vi "Handle getAll.vi"(8 "error in (no error)":errorcluster, 11 "Temperhum":refnum<class "Instrument.Temperhum.lvclass">) -> (0 "error out":errorcluster, 2 "getAll":variant, 3 "Instrument.FrameworkTemplate out":refnum<class "Instrument.Temperhum.lvclass">)   [LabVIEW 2019, in "Instrument.Temperhum.lvclass"]
uses:
  Instrument.Temperhum.lvclass
  Typedefs/Instrument.Temperhum.getAll--Cluster.ctl
  Instrument.Temperhum.lvclass/Instrument.Temperhum.ctl
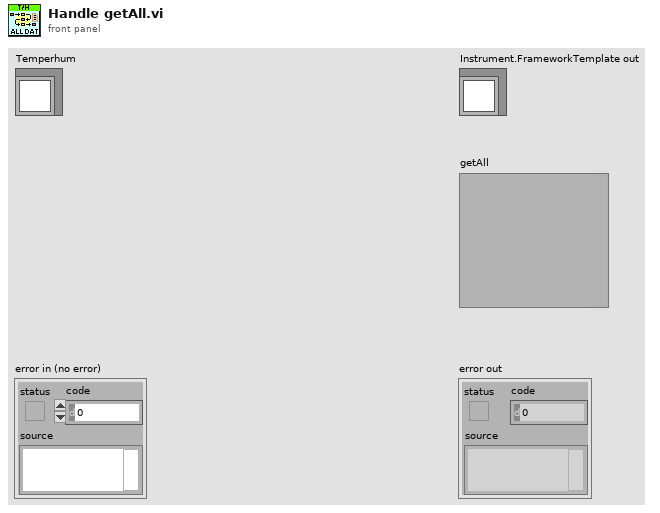
[diagram p1: front panel]
types:
  T1 = typedef "Instrument.Temperhum.lvclass/Instrument.Temperhum.getAll--Cluster.ctl" = cluster{"Temperature (K)":dbl, "Humidity (%RH)":dbl}
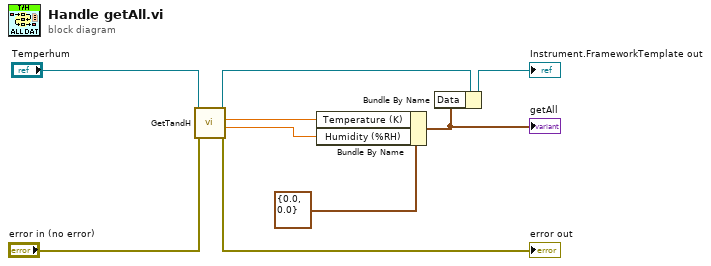
[diagram p0: block diagram]
diagram:
  n1 = call-dynamic "GetTandH.vi"("error in (no error)"="error in (no error)", "Instrument.Temperhum in"="Temperhum") -> ("error out"=→"error out":errorcluster, "Humidity (%RH)"=w7:dbl, "Temperature (K)"=w8:dbl, "Instrument.Temperhum out"=w4:refnum<class "Instrument.Temperhum.lvclass">)  [unwired: 6 in]
  n2 = Bundle By Name(cluster=T1 {"Temperature (K)"=0.0, "Humidity (%RH)"=0.0} ("getAll"), "Temperature (K)"=w8, "Humidity (%RH)"=w7) -> (w1:T1)
  "getAll" <- w1
  n3 = Bundle By Name(cluster=w4, "Data"=w1) -> (→"Instrument.FrameworkTemplate out":refnum<class "Instrument.Temperhum.lvclass">)
